vi "Read Driver Jostick.vi"(11 "Driver Joystick":T1) -> ()   [LabVIEW 2020]
uses:
  <vilib>/Rock Robotics/WPI/Joystick/WPI_JoystickDeviceEnum.ctl
  <vilib>/Rock Robotics/WPI/Joystick/WPI_JoystickDevRef.ctl
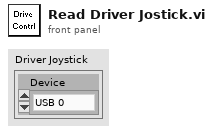
[diagram p1: front panel]
types:
  T1 = typedef "WPI_JoystickDevRef.ctl" = cluster{"Device":T2}
  T2 = typedef "WPI_JoystickDeviceEnum.ctl" = enum16{"USB 0", "USB 1", "USB 2", "USB 3", "USB 4", "USB 5"}
  T3 = enum16{"Left Stick 0: X Axis", "Left Stick 1: Y Axis", "Right Stick 2: Z Axis", "Right Stick 3: Z Rotates"}
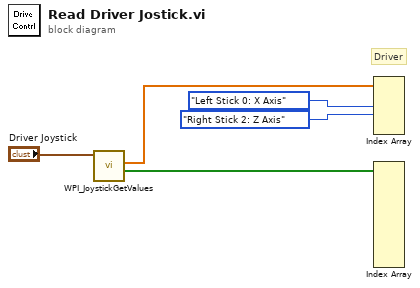
[diagram p0: block diagram]
diagram:
  # "Driver"
  n1 = call <vilib>:"WPI_JoystickGetValues.vi"("JoystickDevRef"="Driver Joystick") -> ("Buttons"=w1:bool[], "Axes"=w4:dbl[])  [unwired: 6 in, 3 out]
  n2 = Index Array(array=w4, index #2=T3."Left Stick 0: X Axis", index #3=T3."Right Stick 2: Z Axis") -> ()  [unwired: 3 in, 5 out]
  n3 = Index Array(array=w1) -> ()  [unwired: 11 in, 11 out]
